vi "SubVI_Save_Impedances_Settings.vi"(8 "error in (no error)":errorcluster) -> (0 "error out":errorcluster)   [LabVIEW 2020]
uses:
  Global 1.vi
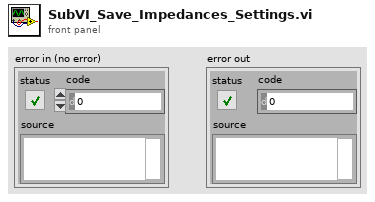
[diagram p1: front panel]
types:
  T1 = enum16{"open", "open or create", "create or replace", "create", "open (read-only)"}
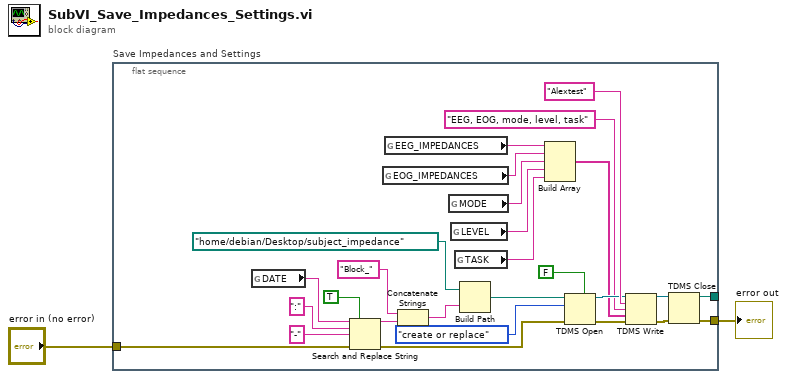
[diagram p0: block diagram]
diagram:
  n1 = flat-sequence "Save Impedances and Settings" {
    tunnel: [w14] -> _
    tunnel: [w13] -> w1
    tunnel: "error in (no error)" -> [w5]
    frame #0 {
      n2 = global read "Global 1.vi" "DATE"() -> (w22:string)
      n3 = Search and Replace String(replace all?=TRUE ("replace all? (F)"), input string=w22, search string=":" ("input string"), replace string="-" ("replace string (\"\")"), error in=w5) -> (result string=w24:string, error out=w4:errorcluster)  [unwired: 3 in, 2 out]
      n4 = global read "Global 1.vi" "EOG_IMPEDANCES"() -> (w12:string)
      n5 = global read "Global 1.vi" "EEG_IMPEDANCES"() -> (w11:string)
      n6 = Concatenate Strings("Block_" ("string"), w24) -> (w27:string)
      n7 = global read "Global 1.vi" "MODE"() -> (w10:string)
      n8 = global read "Global 1.vi" "LEVEL"() -> (w9:string)
      n9 = global read "Global 1.vi" "TASK"() -> (w8:string)
      n10 = Build Path(base path=path "/home/debian/Desktop/subject_impedance", name or relative path=w27) -> (appended path=w3:path)
      n11 = Build Array(w11, w12, w10, w9, w8) -> (w7:string[])
      n12 = TDMS Open(5:FALSE ("create index file? (T)"), 8:w4, 10:T1."create or replace" ("operation (0:open)"), 11:w3) -> (0:w16:errorcluster, 3:w18:refnum<k34>)  [unwired: 3 in]
      n13 = TDMS Write(0:w18, 5:"Alextest" ("group name in (Untitled)"), 7:"EEG, EOG, mode, level, task" ("channel name(s) in (Untitled)"), 9:w7, 11:w16) -> (4:w20:refnum<k34>, 15:w15:errorcluster)  [unwired: 1 in, 2 out]
      n14 = TDMS Close(8:w15, 11:w20) -> (0:w13:errorcluster, 3:w14:path)
    }
  }
  "error out" <- w1
